vi "write_attributes.vi"(8 "error in (no error)":errorcluster caption="entrée d'erreur (pas d'erreur)", 10 "attributes":T1, 11 "FactorAnalysis en entrée":refnum<class "FactorAnalysis.lvclass">) -> (0 "error out":errorcluster caption="sortie d'erreur", 3 "FactorAnalysis en sortie":refnum<class "FactorAnalysis.lvclass">)   [LabVIEW 2020, in "FactorAnalysis.lvclass"]
uses:
  FactorAnalysis.lvclass
  Controls/factor_analysis_attributes.ctl
  FactorAnalysis.lvclass/FactorAnalysis.ctl
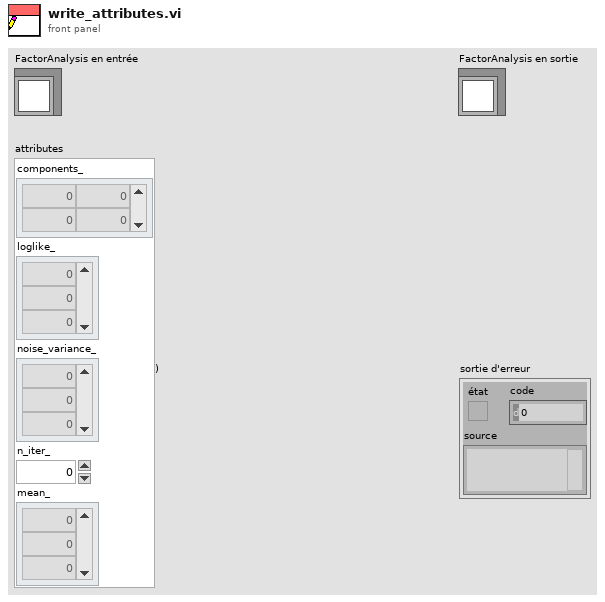
[diagram p1: front panel]
types:
  T1 = typedef "factor_analysis_attributes.ctl" = cluster{"components_":dbl[][], "loglike_":dbl[], "noise_variance_":dbl[], "n_iter_":dbl, "mean_":dbl[]}
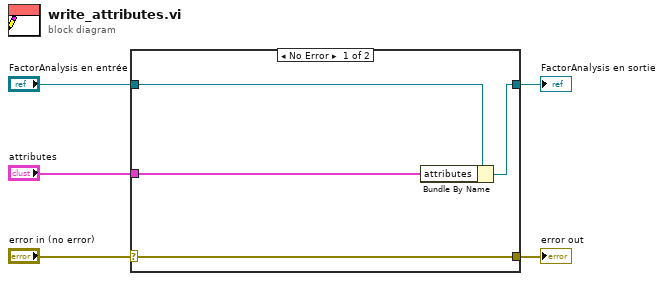
[diagram p0: block diagram]
diagram:
  n1 = case shown="No Error" "error in (no error)" {
    selector: "error in (no error)" -> [w9 w10]
    tunnel: [w9 w10] -> w4
    tunnel: [w7 w11] -> w2
    tunnel: "FactorAnalysis en entrée" -> [w8 w11]
    tunnel: "attributes" -> [w6 _]
    frame No Error {
      n2 = Bundle By Name(cluster=w8, "attributes"=w6) -> (w7:refnum<class "FactorAnalysis.lvclass">)
    }
    frame Error {
    }
  }
  "error out" <- w4
  "FactorAnalysis en sortie" <- w2
